vi "VoltageAdquisition.vi"() -> ()   [LabVIEW 2011]
panel:
  out "Waveform Graph":dynamicdata(graph)
  in  "stop":bool
  out "data":dynamicdata(graph)
  in  "Slide":dbl(slide) scale=0.0..9.0
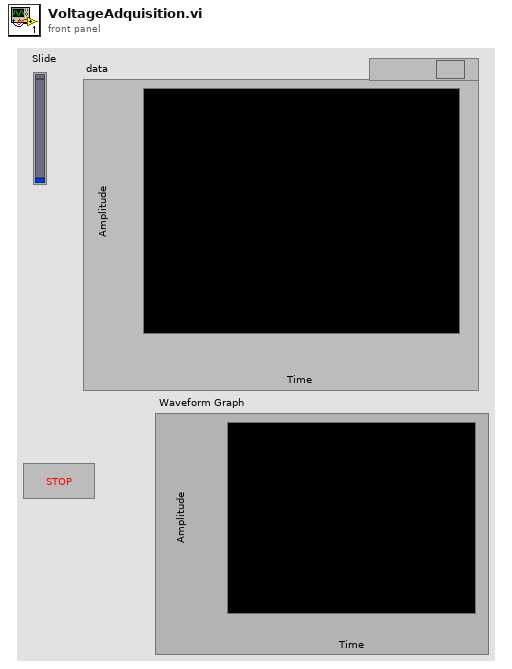
[diagram p1: front panel]
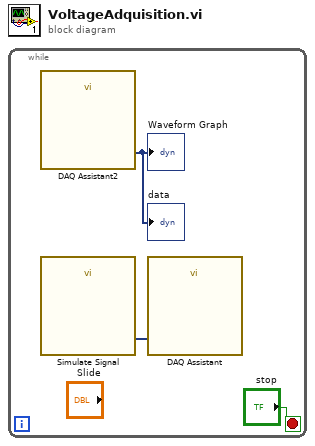
[diagram p0: block diagram]
diagram:
  n1 = while {
    stop <- "stop" stop-if-true
    n2 = call "DAQ Assistant2"() -> ("data"=→"data" →"Waveform Graph":dynamicdata)  [unwired: 17 in, 2 out]
    n3 = call "Simulate Signal"() -> ("Sine"=w2:dynamicdata)  [unwired: 14 in, 1 out]
    n4 = call "DAQ Assistant"("data"=w2) -> ()  [unwired: 17 in, 2 out]
  }
